vi "Shortcuts.vi"() -> (3 "Modbus Shortcuts":T1[](array[typedef]))   [LabVIEW 2020, in "Modbus.lvlib" / "Modbus.lvclass"]
uses:
  Modbus.lvclass
  Modbus Control Shortcut.ctl
  Modbus Channel Type.ctl
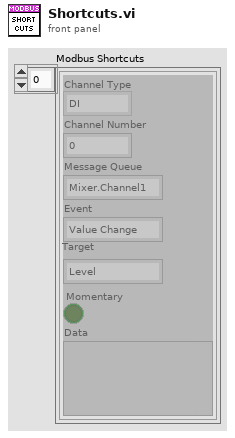
[diagram p1: front panel]
types:
  T1 = typedef "Modbus.lvlib/Modbus.lvclass/Modbus Control Shortcut.ctl" = cluster{"Channel Type":T2, "Channel Number":u8, "Message Queue":string, "Event":string, "Target":string, "Momentary":bool, "Data":variant}
  T2 = typedef "Modbus.lvlib/Modbus.lvclass/Modbus Channel Type.ctl" = enum16{"DI", "AI"}
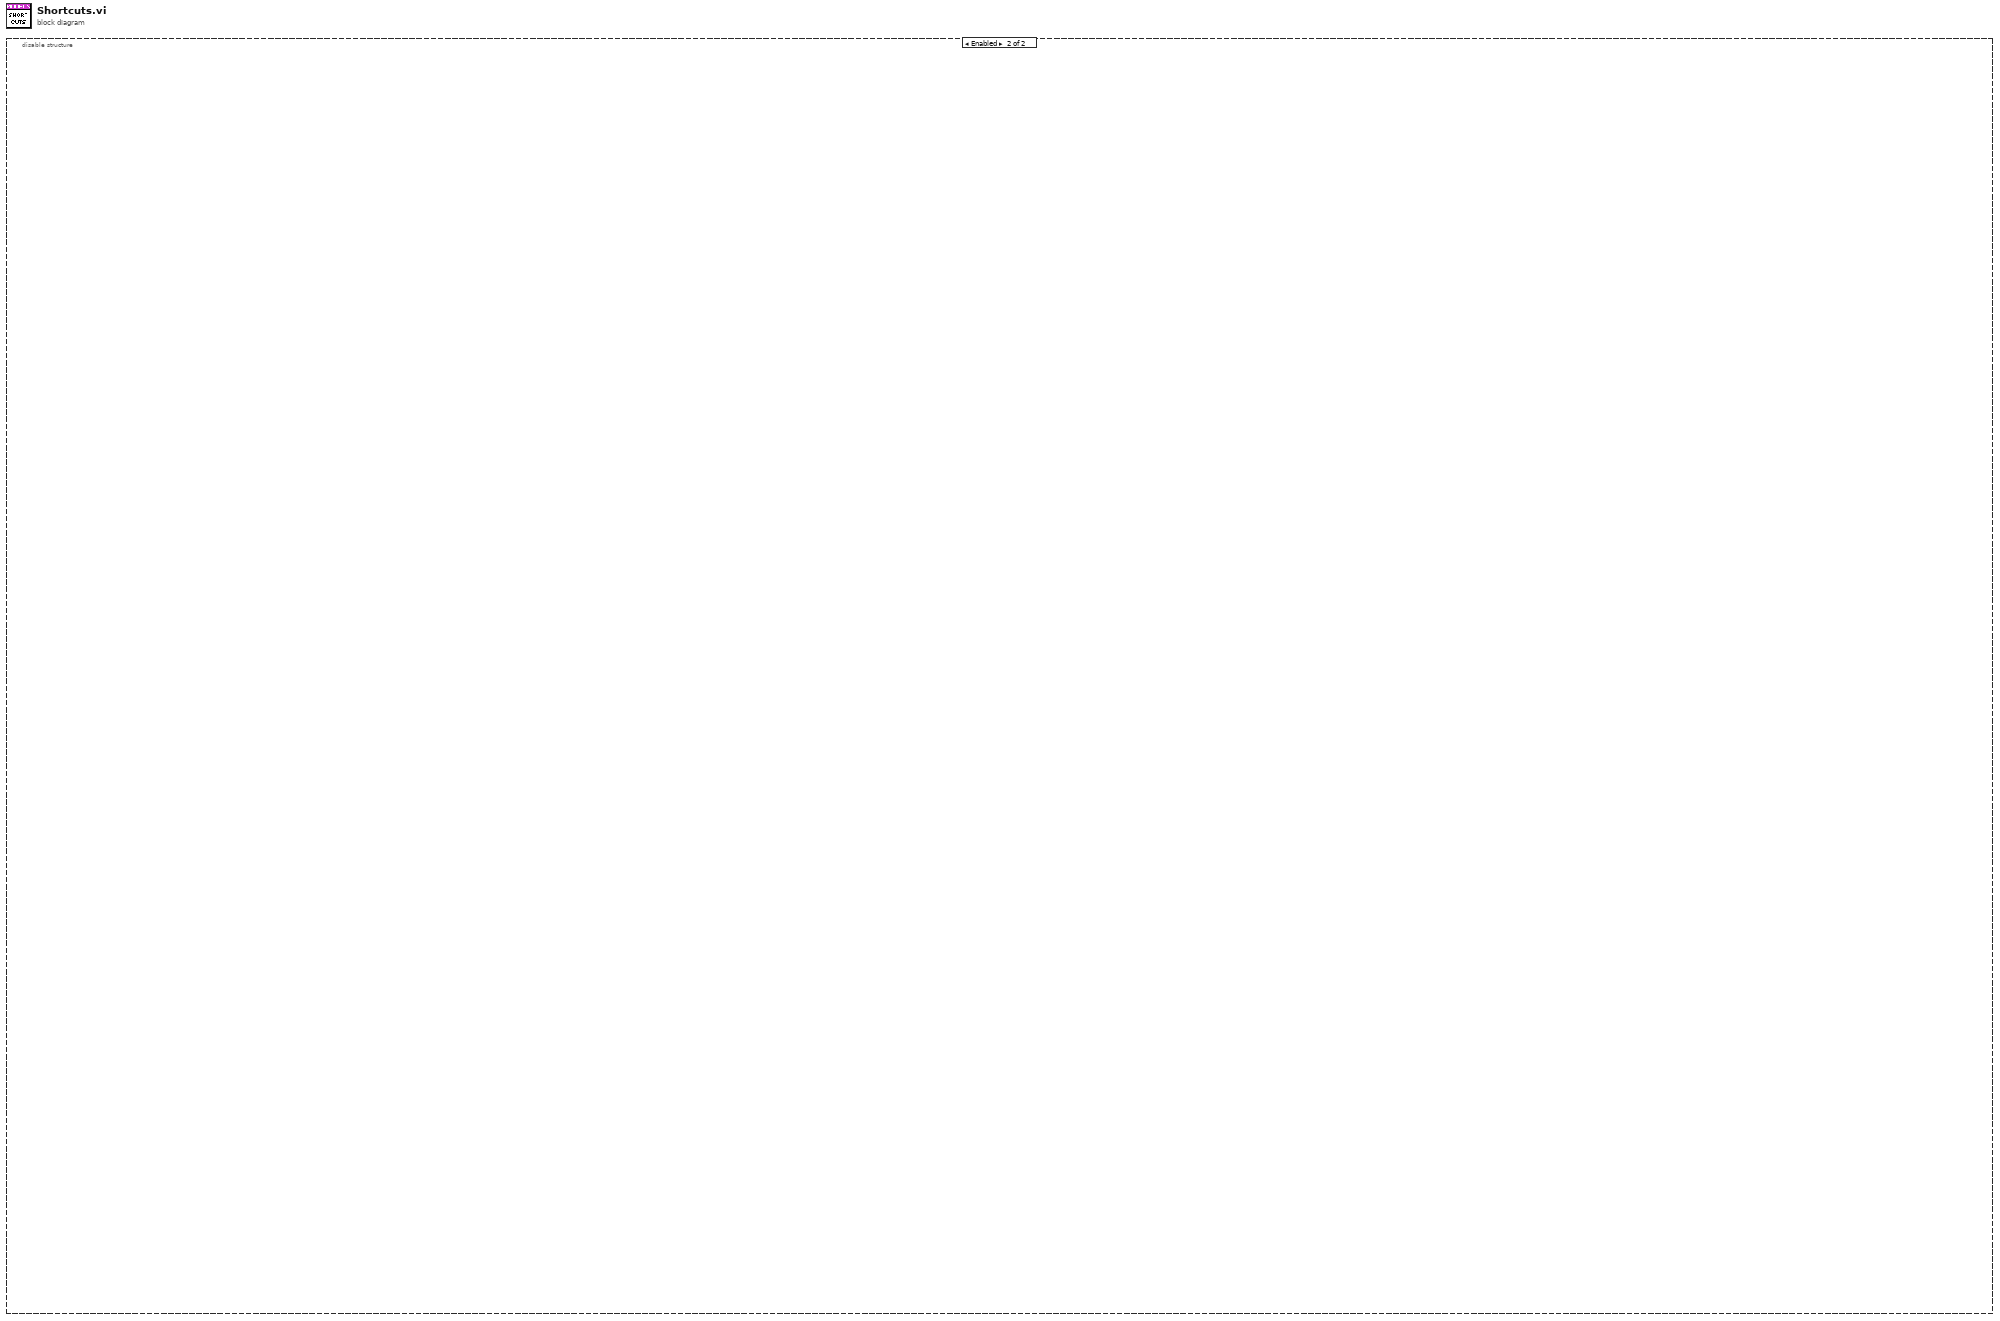
[diagram p0: block diagram]
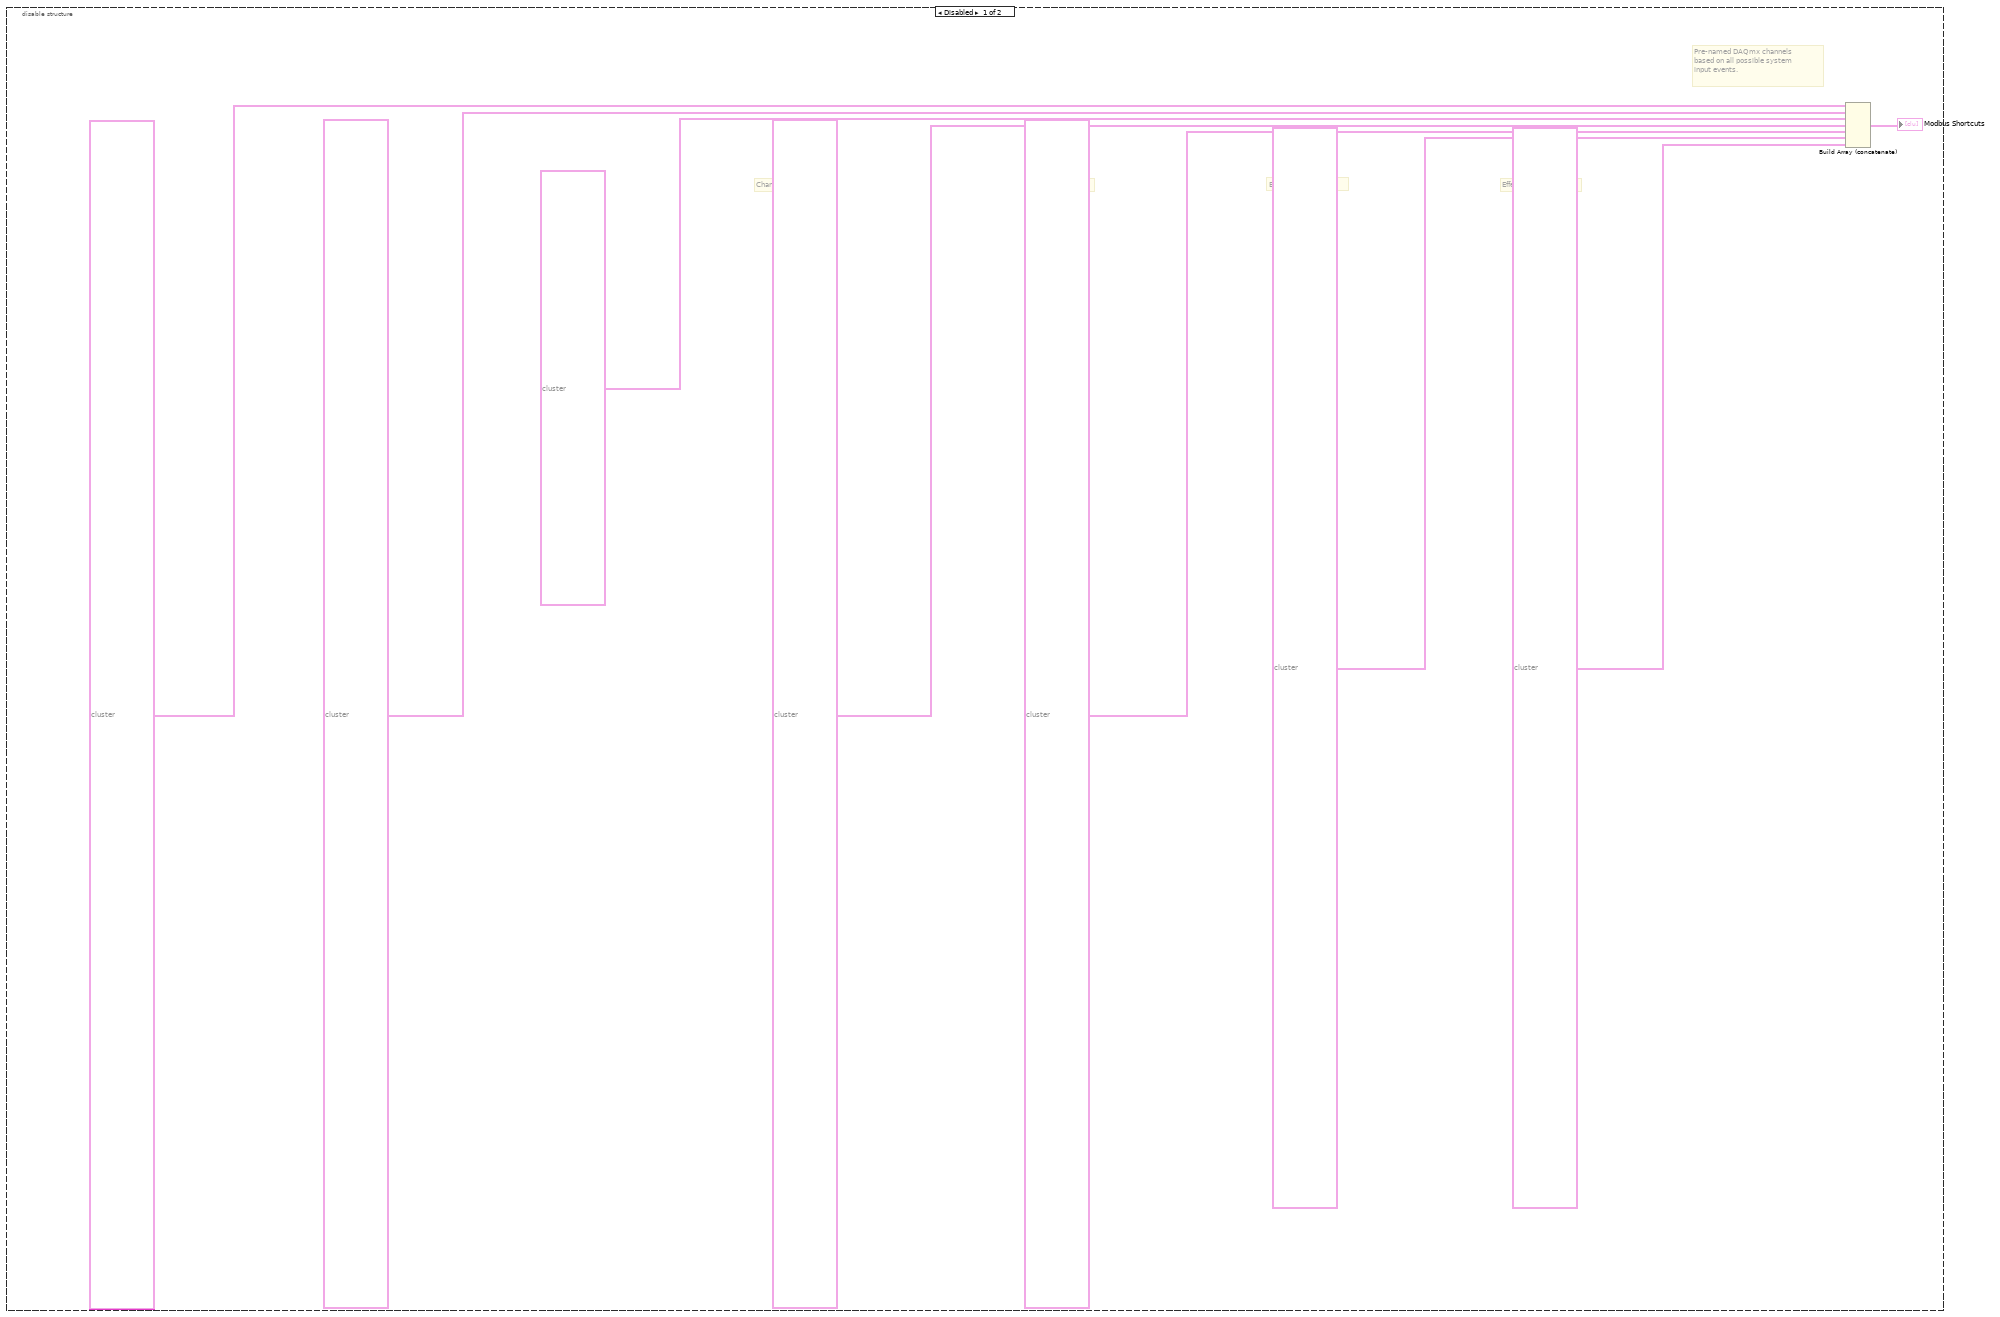
[diagram p2: hidden frame]
diagram:
  n1 = disable-structure shown="Enabled" {
    frame Disabled {
      # "Deck2"
      # "Deck1"
      # "EffectUnit2.Effectn"
      # "EffectUnit1.Effectn"
      # "Channel2"
      # "Channel1"
      # "Mixer"
      # "Pre-named DAQmx channels based on all possible system input events."
      n2 = Build Array (concatenate)(T1[] [{"Channel Type"=enum."DI", "Channel Number"=0, "Message Queue"="Deck1", "Event"="Toggle", "Target"="Play", "Momentary"=FALSE, "Data"=variant}, {"Channel Type"=enum."DI", "Channel Number"=0, "Message Queue"="Deck1", "Event"="Toggle", "Target"="Brake", "Momentary"=FALSE, "Data"=variant}, {"Channel Type"=enum."DI", "Channel Number"=0, "Message Queue"="Deck1", "Event"="Toggle", "Target"="Backspin", "Momentary"=FALSE, "Data"=variant}, {"Channel Type"=enum."DI", "Channel Number"=0, "Message Queue"="Deck1", "Event"="Toggle", "Target"="Reverse", "Momentary"=FALSE, "Data"=variant}, {"Channel Type"=enum."DI", "Channel Number"=0, "Message Queue"="Deck1", "Event"="Value Change", "Target"="Cue1", "Momentary"=FALSE, "Data"=variant}, {"Channel Type"=enum."DI", "Channel Number"=0, "Message Queue"="Deck1", "Event"="Value Change", "Target"="Cue2", "Momentary"=FALSE, "Data"=variant}, {"Channel Type"=enum."DI", "Channel Number"=0, "Message Queue"="Deck1", "Event"="Value Change", "Target"="Cue3", "Momentary"=FALSE, "Data"=variant}, {"Channel Type"=enum."DI", "Channel Number"=0, "Message Queue"="Deck1", "Event"="Value Change", "Target"="PitchBendDown", "Momentary"=TRUE, "Data"=variant}, {"Channel Type"=enum."DI", "Channel Number"=0, "Message Queue"="Deck1", "Event"="Value Change", "Target"="PitchBendUp", "Momentary"=TRUE, "Data"=variant}, {"Channel Type"=enum."DI", "Channel Number"=0, "Message Queue"="Deck1", "Event"="Value Change", "Target"="Pitch", "Momentary"=FALSE, "Data"=variant}], T1[] [{"Channel Type"=enum."DI", "Channel Number"=0, "Message Queue"="Deck2", "Event"="Toggle", "Target"="Play", "Momentary"=FALSE, "Data"=variant}, {"Channel Type"=enum."DI", "Channel Number"=0, "Message Queue"="Deck2", "Event"="Toggle", "Target"="Brake", "Momentary"=FALSE, "Data"=variant}, {"Channel Type"=enum."DI", "Channel Number"=0, "Message Queue"="Deck2", "Event"="Toggle", "Target"="Backspin", "Momentary"=FALSE, "Data"=variant}, {"Channel Type"=enum."DI", "Channel Number"=0, "Message Queue"="Deck2", "Event"="Toggle", "Target"="Reverse", "Momentary"=FALSE, "Data"=variant}, {"Channel Type"=enum."DI", "Channel Number"=0, "Message Queue"="Deck2", "Event"="Value Change", "Target"="Cue1", "Momentary"=FALSE, "Data"=variant}, {"Channel Type"=enum."DI", "Channel Number"=0, "Message Queue"="Deck2", "Event"="Value Change", "Target"="Cue2", "Momentary"=FALSE, "Data"=variant}, {"Channel Type"=enum."DI", "Channel Number"=0, "Message Queue"="Deck2", "Event"="Value Change", "Target"="Cue3", "Momentary"=FALSE, "Data"=variant}, {"Channel Type"=enum."DI", "Channel Number"=0, "Message Queue"="Deck2", "Event"="Value Change", "Target"="PitchBendDown", "Momentary"=TRUE, "Data"=variant}, {"Channel Type"=enum."DI", "Channel Number"=0, "Message Queue"="Deck2", "Event"="Value Change", "Target"="PitchBendUp", "Momentary"=TRUE, "Data"=variant}, {"Channel Type"=enum."DI", "Channel Number"=0, "Message Queue"="Deck2", "Event"="Value Change", "Target"="Pitch", "Momentary"=FALSE, "Data"=variant}], T1[] [{"Channel Type"=enum."DI", "Channel Number"=0, "Message Queue"="Mixer", "Event"="Value Change", "Target"="Master", "Momentary"=FALSE, "Data"=variant}, {"Channel Type"=enum."DI", "Channel Number"=0, "Message Queue"="Mixer", "Event"="Value Change", "Target"="Headphones", "Momentary"=FALSE, "Data"=variant}, {"Channel Type"=enum."DI", "Channel Number"=0, "Message Queue"="Mixer", "Event"="Value Change", "Target"="Crossfader", "Momentary"=FALSE, "Data"=variant}], T1[] [{"Channel Type"=enum."DI", "Channel Number"=0, "Message Queue"="Channel1", "Event"="Value Change", "Target"="Gain", "Momentary"=FALSE, "Data"=variant}, {"Channel Type"=enum."DI", "Channel Number"=0, "Message Queue"="Channel1", "Event"="Value Change", "Target"="Level", "Momentary"=FALSE, "Data"=variant}, {"Channel Type"=enum."DI", "Channel Number"=0, "Message Queue"="Channel1", "Event"="Value Change", "Target"="EQHigh", "Momentary"=FALSE, "Data"=variant}, {"Channel Type"=enum."DI", "Channel Number"=0, "Message Queue"="Channel1", "Event"="Value Change", "Target"="EQMid", "Momentary"=FALSE, "Data"=variant}, {"Channel Type"=enum."DI", "Channel Number"=0, "Message Queue"="Channel1", "Event"="Value Change", "Target"="EQLow", "Momentary"=FALSE, "Data"=variant}, {"Channel Type"=enum."DI", "Channel Number"=0, "Message Queue"="Channel1", "Event"="Value Change", "Target"="EQFilter", "Momentary"=FALSE, "Data"=variant}, {"Channel Type"=enum."DI", "Channel Number"=0, "Message Queue"="Channel1", "Event"="Toggle", "Target"="EQHighKill", "Momentary"=FALSE, "Data"=variant}, {"Channel Type"=enum."DI", "Channel Number"=0, "Message Queue"="Channel1", "Event"="Toggle", "Target"="EQMidKill", "Momentary"=FALSE, "Data"=variant}, {"Channel Type"=enum."DI", "Channel Number"=0, "Message Queue"="Channel1", "Event"="Toggle", "Target"="EQLowKill", "Momentary"=FALSE, "Data"=variant}, {"Channel Type"=enum."DI", "Channel Number"=0, "Message Queue"="Channel1", "Event"="Toggle", "Target"="HeadphoneOutput", "Momentary"=FALSE, "Data"=variant}], T1[] [{"Channel Type"=enum."DI", "Channel Number"=0, "Message Queue"="Channel2", "Event"="Value Change", "Target"="Gain", "Momentary"=FALSE, "Data"=variant}, {"Channel Type"=enum."DI", "Channel Number"=0, "Message Queue"="Channel2", "Event"="Value Change", "Target"="Level", "Momentary"=FALSE, "Data"=variant}, {"Channel Type"=enum."DI", "Channel Number"=0, "Message Queue"="Channel2", "Event"="Value Change", "Target"="EQHigh", "Momentary"=FALSE, "Data"=variant}, {"Channel Type"=enum."DI", "Channel Number"=0, "Message Queue"="Channel2", "Event"="Value Change", "Target"="EQMid", "Momentary"=FALSE, "Data"=variant}, {"Channel Type"=enum."DI", "Channel Number"=0, "Message Queue"="Channel2", "Event"="Value Change", "Target"="EQLow", "Momentary"=FALSE, "Data"=variant}, {"Channel Type"=enum."DI", "Channel Number"=0, "Message Queue"="Channel2", "Event"="Value Change", "Target"="EQFilter", "Momentary"=FALSE, "Data"=variant}, {"Channel Type"=enum."DI", "Channel Number"=0, "Message Queue"="Channel2", "Event"="Toggle", "Target"="EQHighKill", "Momentary"=FALSE, "Data"=variant}, {"Channel Type"=enum."DI", "Channel Number"=0, "Message Queue"="Channel2", "Event"="Toggle", "Target"="EQMidKill", "Momentary"=FALSE, "Data"=variant}, {"Channel Type"=enum."DI", "Channel Number"=0, "Message Queue"="Channel2", "Event"="Toggle", "Target"="EQLowKill", "Momentary"=FALSE, "Data"=variant}, {"Channel Type"=enum."DI", "Channel Number"=0, "Message Queue"="Channel2", "Event"="Toggle", "Target"="HeadphoneOutput", "Momentary"=FALSE, "Data"=variant}], T1[] [{"Channel Type"=enum."DI", "Channel Number"=0, "Message Queue"="EffectUnit1.Effect1", "Event"="Value Change", "Target"="Value1", "Momentary"=FALSE, "Data"=variant}, {"Channel Type"=enum."DI", "Channel Number"=0, "Message Queue"="EffectUnit1.Effect1", "Event"="Value Change", "Target"="Value2", "Momentary"=FALSE, "Data"=variant}, {"Channel Type"=enum."DI", "Channel Number"=0, "Message Queue"="EffectUnit1.Effect1", "Event"="Toggle", "Target"="Enable", "Momentary"=FALSE, "Data"=variant}, {"Channel Type"=enum."DI", "Channel Number"=0, "Message Queue"="EffectUnit1.Effect2", "Event"="Value Change", "Target"="Value1", "Momentary"=FALSE, "Data"=variant}, {"Channel Type"=enum."DI", "Channel Number"=0, "Message Queue"="EffectUnit1.Effect2", "Event"="Value Change", "Target"="Value2", "Momentary"=FALSE, "Data"=variant}, {"Channel Type"=enum."DI", "Channel Number"=0, "Message Queue"="EffectUnit1.Effect2", "Event"="Toggle", "Target"="Enable", "Momentary"=FALSE, "Data"=variant}, {"Channel Type"=enum."DI", "Channel Number"=0, "Message Queue"="EffectUnit1.Effect3", "Event"="Value Change", "Target"="Value1", "Momentary"=FALSE, "Data"=variant}, {"Channel Type"=enum."DI", "Channel Number"=0, "Message Queue"="EffectUnit1.Effect3", "Event"="Value Change", "Target"="Value2", "Momentary"=FALSE, "Data"=variant}, {"Channel Type"=enum."DI", "Channel Number"=0, "Message Queue"="EffectUnit1.Effect3", "Event"="Toggle", "Target"="Enable", "Momentary"=FALSE, "Data"=variant}], T1[] [{"Channel Type"=enum."DI", "Channel Number"=0, "Message Queue"="EffectUnit2.Effect1", "Event"="Value Change", "Target"="Value1", "Momentary"=FALSE, "Data"=variant}, {"Channel Type"=enum."DI", "Channel Number"=0, "Message Queue"="EffectUnit2.Effect1", "Event"="Value Change", "Target"="Value2", "Momentary"=FALSE, "Data"=variant}, {"Channel Type"=enum."DI", "Channel Number"=0, "Message Queue"="EffectUnit2.Effect1", "Event"="Toggle", "Target"="Enable", "Momentary"=FALSE, "Data"=variant}, {"Channel Type"=enum."DI", "Channel Number"=0, "Message Queue"="EffectUnit2.Effect2", "Event"="Value Change", "Target"="Value1", "Momentary"=FALSE, "Data"=variant}, {"Channel Type"=enum."DI", "Channel Number"=0, "Message Queue"="EffectUnit2.Effect2", "Event"="Value Change", "Target"="Value2", "Momentary"=FALSE, "Data"=variant}, {"Channel Type"=enum."DI", "Channel Number"=0, "Message Queue"="EffectUnit2.Effect2", "Event"="Toggle", "Target"="Enable", "Momentary"=FALSE, "Data"=variant}, {"Channel Type"=enum."DI", "Channel Number"=0, "Message Queue"="EffectUnit2.Effect3", "Event"="Value Change", "Target"="Value1", "Momentary"=FALSE, "Data"=variant}, {"Channel Type"=enum."DI", "Channel Number"=0, "Message Queue"="EffectUnit2.Effect3", "Event"="Value Change", "Target"="Value2", "Momentary"=FALSE, "Data"=variant}, {"Channel Type"=enum."DI", "Channel Number"=0, "Message Queue"="EffectUnit2.Effect3", "Event"="Toggle", "Target"="Enable", "Momentary"=FALSE, "Data"=variant}]) -> (→"Modbus Shortcuts":T1[])
    }
    frame Enabled {
    }
  }
